vi "KE622x -- Set Source Delay.vi"(0 "Resource In":refnum<visa-resource-name>, 1 "Check For SCPI Errors? (T)":bool=TRUE, 7 "Source Delay (s)":dbl=1.0 min=0.001 max=1000.0 step=0.001 format="%.3f", 11 "error in (no error)":errorcluster) -> (4 "Resource Out (dupl)":refnum<visa-resource-name>, 15 "error out":errorcluster)   [LabVIEW 2013, in "Keithly user program.lvlib"]
doc: "Sets the settling time (a.k.a. 'source delay') for all steps in a current sweep."
uses:
  Keithly user program.lvlib
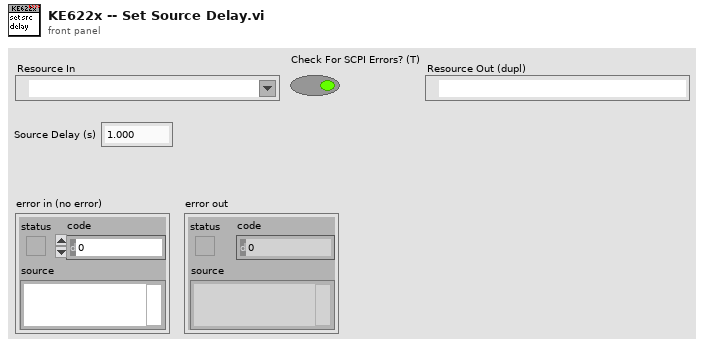
[diagram p1: front panel]
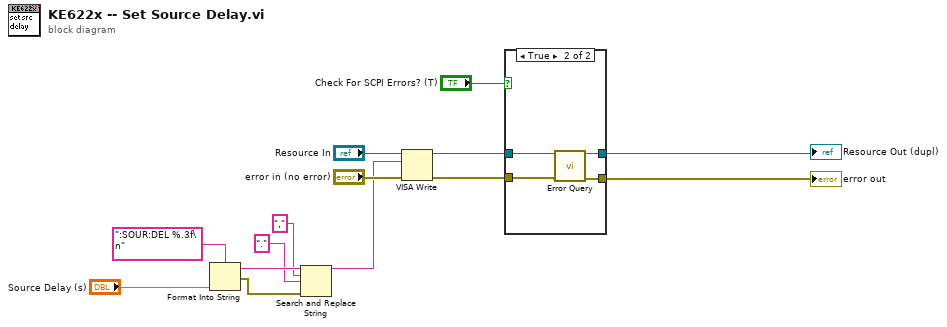
[diagram p0: block diagram]
diagram:
  n1 = Format Into String(format string=":SOUR:DEL %.3f\n", "Source Delay (s)") -> (resulting string=w5:string, error out=w4:errorcluster)  [unwired: 2 in]
  n2 = Search and Replace String(input string=w5, search string=",", replace string="." ("replace string (\"\")"), error in=w4) -> (result string=w3:string)  [unwired: 4 in, 3 out]
  n3 = VISA Write(VISA resource name="Resource In", write buffer=w3, error in (no error)="error in (no error)") -> (VISA resource name out=w10:refnum<visa-resource-name>, error out=w9:errorcluster)  [unwired: 1 out]
  n4 = case shown="True" "Check For SCPI Errors? (T)" {
    tunnel: w10 -> [w16 w20]
    tunnel: w9 -> [w15 w17]
    tunnel: [w15 w18] -> w7
    tunnel: [w16 w19] -> w8
    frame False {
    }
    frame True {
      n5 = call "Error Query.vi"("VISA Resource In"=w20, "error in (no error)"=w17) -> ("VISA Resource Out (dupl)"=w19:refnum<visa-resource-name>, "error out"=w18:errorcluster)  [unwired: 10 in, 2 out]
    }
  }
  "Resource Out (dupl)" <- w8
  "error out" <- w7
